vi "Stop.vi"(8 "error in":errorcluster, 11 "DO DAQmx PWM Fixed Freq CFG in":refnum<class "DO DAQmx PWM Fixed Freq CFG.lvclass">) -> (0 "error out":errorcluster, 3 "DO DAQmx PWM Fixed Freq CFG out":refnum<class "DO DAQmx PWM Fixed Freq CFG.lvclass">)   [LabVIEW 2023, in "DAQmx Simulated CFGs.lvlib" / "DO DAQmx PWM Fixed Freq CFG.lvclass"]
uses:
  DO DAQmx PWM Fixed Freq CFG.lvclass
  DO DAQmx PWM Fixed Freq CFG.lvclass/DO DAQmx PWM Fixed Freq CFG.ctl
  DO DAQmx Fixed Freq PWM CFG/DO DAQmx Fixed Freq PWM CFG.lvclass
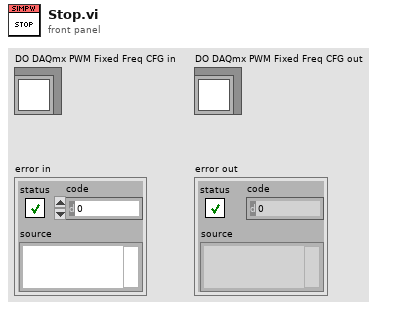
[diagram p1: front panel]
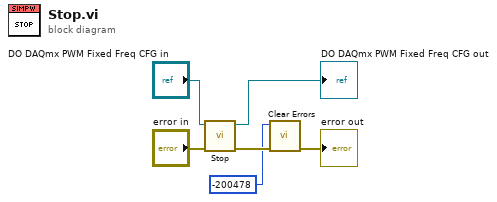
[diagram p0: block diagram]
diagram:
  n1 = call-parent "Stop.vi"("error in"="error in", "DAQmx Base CFG in"="DO DAQmx PWM Fixed Freq CFG in") -> ("error out"=w6:errorcluster, "DAQmx Base CFG out"=→"DO DAQmx PWM Fixed Freq CFG out":refnum<class "DO DAQmx PWM Fixed Freq CFG.lvclass">)  [unwired: 8 in]
  n2 = call <vilib>:"Clear Errors.vi"("error in (no error)"=w6, "specific error code to clear (0: all)"=-200478) -> ("error out"=→"error out":errorcluster)  [unwired: 4 in, 1 out]
